vi "Throw Invalid Step Error.vi"(6 "Step Number":i32, 7 "Num Steps":i32, 8 "error in (no error)":errorcluster, 11 "Action String in":string) -> (0 "error out":errorcluster)   [LabVIEW 2024, in "Output Sequencer.lvlib" / "Output Sequencer.lvclass"]
uses:
  Output Sequencer.lvclass
  Globals/Global Strings.vi
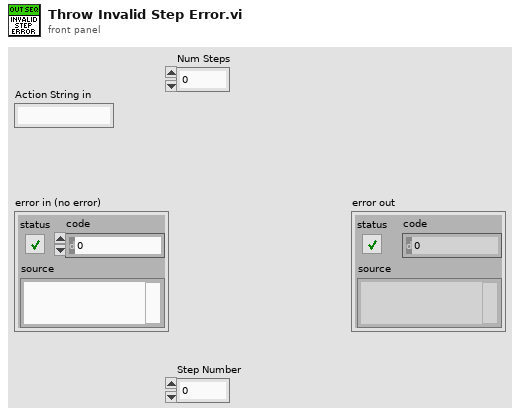
[diagram p1: front panel]
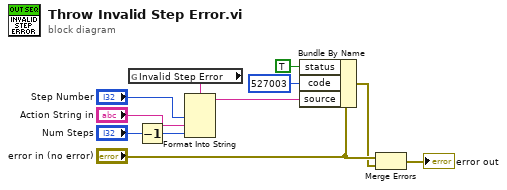
[diagram p0: block diagram]
diagram:
  n1 = global read "Global Strings.vi" "Invalid Step Error"() -> (w11:string)
  n2 = Decrement(x="Num Steps") -> (x-1=w1:i32)
  n3 = Format Into String(format string=w11, "Step Number", "Action String in", w1) -> (resulting string=w10:string)  [unwired: 2 in, 1 out]
  n4 = Bundle By Name(cluster="error in (no error)", "status"=TRUE ("is warning? (False)"), "code"=527003 ("error code (0)"), "source"=w10) -> (w6:errorcluster)
  n5 = Merge Errors("error in (no error)", w6) -> (→"error out":errorcluster)
